vi "Read Setup File.lvclass.vi"(8 "error in (no error)":errorcluster, 11 "SPARC4_AC in":refnum<class "S4GUI.lvclass">) -> (0 "error out":errorcluster, 2 "Setup File.lvclass":refnum<class "Setup File.lvclass">, 3 "SPARC4_AC out":refnum<class "S4GUI.lvclass">)   [LabVIEW 2018, in "S4GUI.lvclass"]
uses:
  S4GUI.lvclass
  SetupFile/Setup File.lvclass
  S4GUI.lvclass/S4GUI.ctl
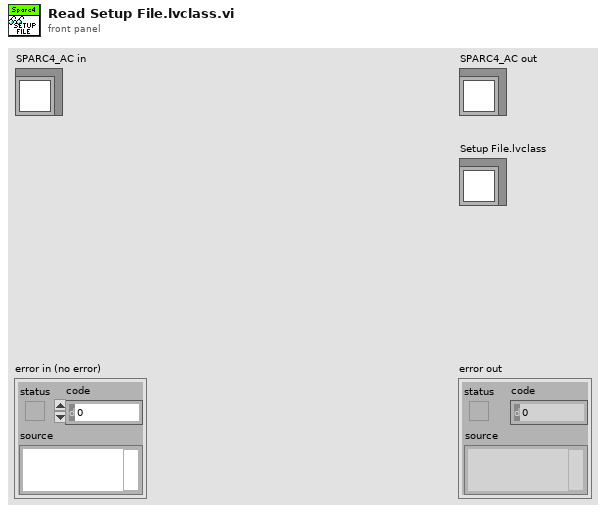
[diagram p1: front panel]
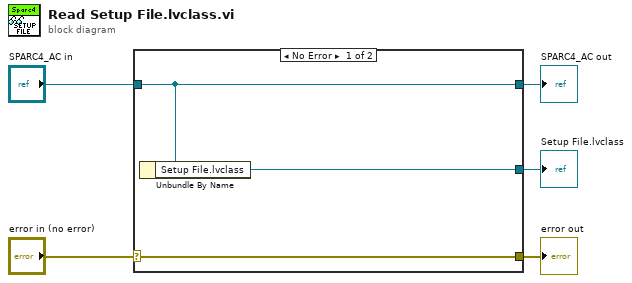
[diagram p0: block diagram]
diagram:
  n1 = case shown="No Error" "error in (no error)" {
    selector: "error in (no error)" -> [w8 w9]
    tunnel: [w8 w9] -> w4
    tunnel: [w7 w10] -> w2
    tunnel: "SPARC4_AC in" -> [w7 w10]
    tunnel: [w6 _] -> w1
    frame No Error {
      n2 = Unbundle By Name(w7) -> ("Setup File.lvclass"=w6:refnum<class "Setup File.lvclass">)
    }
    frame Error {
    }
  }
  "error out" <- w4
  "SPARC4_AC out" <- w2
  "Setup File.lvclass" <- w1
